vi "Finalize.vi"(8 "error in":errorcluster, 11 "Ballard ARINC-429 shared resources in":refnum<class "Ballard ARINC-429 Shared Resources.lvclass">) -> (0 "error out":errorcluster, 3 "Ballard ARINC-429 shared resources out":refnum<class "Ballard ARINC-429 Shared Resources.lvclass">)   [LabVIEW 2020, in "Ballard ARINC 429 Engine.lvlib" / "Implementation.lvlib" / "Ballard ARINC-429 Shared Resources.lvclass"]
uses:
  Ballard ARINC-429 Shared Resources.lvclass
  Ballard ARINC-429 Shared Resources.lvclass/Ballard ARINC-429 Shared Resources.ctl
  Custom Device/Hardware Handles.ctl
  Custom Device/Custom Device.lvlib
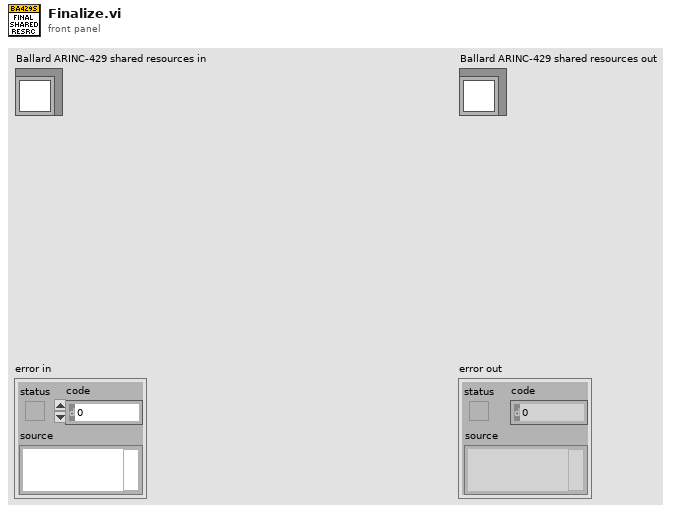
[diagram p1: front panel]
types:
  T1 = typedef "Ballard ARINC 429 Engine.lvlib/Custom Device.lvlib/Hardware Handles.ctl" = cluster{"core handle":u64, "core reader handle":u64, "channel handles":u64[]}
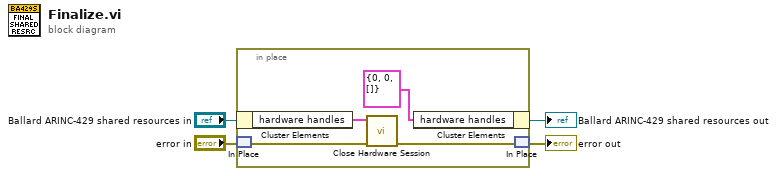
[diagram p0: block diagram]
diagram:
  n1 = in-place {
    n2 = in-place-cluster #1("Ballard ARINC-429 shared resources in") -> ("hardware handles"=w8:T1)
    n3 = in-place-match #2("error in") -> (w7:errorcluster)
    n4 = call "Close Hardware Session.vi"("error in"=w7, "hardware handles"=w8) -> ("error out"=w6:errorcluster)  [unwired: 9 in]
    n5 = in-place-cluster #1("hardware handles"=T1 {"core handle"=0, "core reader handle"=0, "channel handles"=[]} ("RT handles")) -> (→"Ballard ARINC-429 shared resources out":refnum<class "Ballard ARINC-429 Shared Resources.lvclass">)
    n6 = in-place-match #2(w6) -> (→"error out":errorcluster)
  }
